vi "test Action Update Ramp Rate-RampRate10.vi"() -> ()   [LabVIEW 2018, in "AllComponentTestes.lvclass"]
uses:
  AllComponentTestes.lvclass
  C:/Program Files/National Instruments/LabVIEW 2018/vi.lib/addons/_JKI Toolkits/VI Tester/TestCase.llb/TestCase.lvclass
  <vilib>/addons/_JKI Toolkits/VI Tester/TestCase.llb/TestCase.lvclass
  Libraries/Thermal Chamber Controller_DQMH/Thermal Chamber Controller_DQMH.lvlib
  Libraries/Thermal Chamber Response Simulator/Thermal Chamber Response Simulator.lvlib
panel:
  out "TestCase out":refnum<class "TestCase.lvclass">
  in  "TestCase in":refnum<class "AllComponentTestes.lvclass">
  out "error out":errorcluster
  in  "error in (no error)":errorcluster
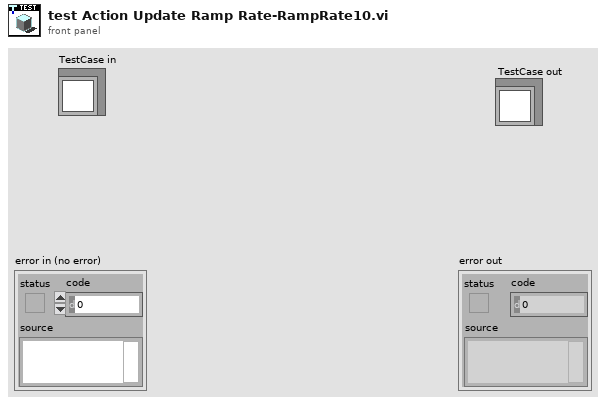
[diagram p1: front panel]
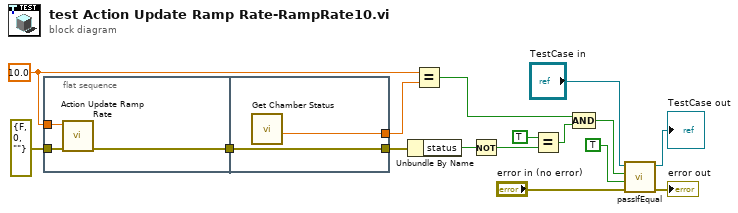
[diagram p0: block diagram]
diagram:
  w1 = 10.0 ("Temperature Set Point")
  n1 = flat-sequence {
    tunnel: errorcluster {"status"=FALSE, "code"=0, "source"=""} ("error in (no error)") -> [w18]
    tunnel: w1 -> [w17]
    tunnel: [w19] -> w16
    tunnel: [w21] -> w5
    tunnel: w16 -> [w21]
    tunnel: [w20] -> w2
    frame #0 {
      n2 = call "Action Update Ramp Rate.vi"("error in (no error)"=w18, "Temperature Ramp Rate"=w17) -> ("error out"=w19:errorcluster)  [unwired: 9 in]
    }
    frame #1 {
      n3 = call "Get Chamber Status.vi"() -> ("Ramp Rate (deg C / second)"=w20:dbl)  [unwired: 6 in, 5 out]
    }
  }
  n4 = Unbundle By Name(w5) -> ("status"=w7:bool)
  n5 = Equal?(x=w1, y=w2) -> (x = y?=w9:bool)
  n6 = Not(x=w7) -> (.not. x?=w6:bool)
  n7 = Equal?(x=TRUE, y=w6) -> (x = y?=w8:bool)
  n8 = Compound Arithmetic op=AND(w9, w8) -> (w4:bool)
  n9 = call-dynamic "passIfEqual.vi"("error in (no error)"="error in (no error)", "y"=TRUE, "x"=w4, "TestCase in"="TestCase in") -> ("error out"=→"error out":errorcluster, "TestCase out"=→"TestCase out":refnum<class "AllComponentTestes.lvclass">)  [unwired: 6 in]
